vi "old_Add To Class.vi"(9 "Ctl Refnum":refnum<vi>, 10 "User VI Ref":refnum<vi>) -> ()   [LabVIEW 2021, in "_Refactor Msg.lvlib" / "Control To Private Data.lvlib"]
uses:
  Control To Private Data.lvlib
  <vilib>/Utility/traverseref.llb/TRef TravTarget.ctl
  <vilib>/Utility/miscctls.llb/LVPositionTypeDef.ctl
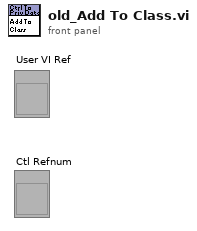
[diagram p1: front panel]
types:
  T1 = typedef "LVPositionTypeDef.ctl" = cluster{"Left":i32, "Top":i32}
  T2 = typedef "TRef TravTarget.ctl" = enum16{"FP", "BD", "Other"}
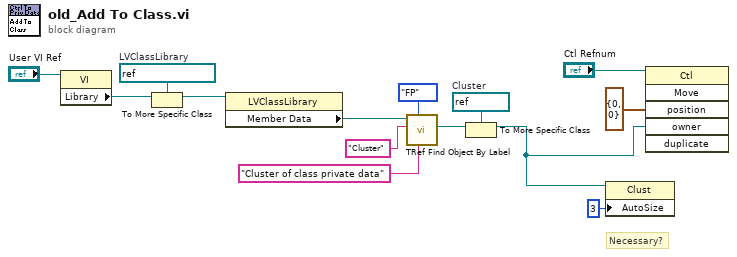
[diagram p0: block diagram]
diagram:
  w5 = refnum<vi> refnum  # Cluster
  w12 = refnum<vi> refnum  # LVClassLibrary
  # "Necessary?"
  n1 = property class="VI"(reference="User VI Ref") -> ("Library"=w13:refnum<vi>)  [unwired: 1 in, 2 out]
  n2 = To More Specific Class(target class=w12, reference=w13) -> (specific class reference=w11:refnum<vi>)  [unwired: 1 in, 1 out]
  n3 = property class="LVClassLibrary"(reference=w11) -> ("Member Data"=w10:refnum<vi>)  [unwired: 1 in, 2 out]
  n4 = call <vilib>:"TRef Find Object By Label.vi"("Label"="Cluster of class private data" ("Class Name"), "Traverse Target"=TRef_TravTarget."FP", "Class Name"="Cluster", "VI Ref"=w10) -> ("Found Obj Ref"=w6:refnum<vi>)  [unwired: 4 in, 3 out]
  n5 = To More Specific Class(target class=w5, reference=w6) -> (specific class reference=w3:refnum<vi>)  [unwired: 1 in, 1 out]
  n6 = property class="Clust"(reference=w3, "AutoSize"=u32 3 ("Auto Sizing")) -> ()  [unwired: 1 in, 2 out]
  n7 = invoke class="Ctl" method="Move"(reference="Ctl Refnum", "position"=T1 {"Left"=0, "Top"=0}, "owner"=w3) -> ()  [unwired: 3 in, 6 out]
